vi "DataHandler Init.vi"(8 "error in (no error)":errorcluster, 11 "DataLogger in":refnum<class "DataLogger.lvclass">) -> (0 "error out":errorcluster, 3 "DataLogger out":refnum<class "DataLogger.lvclass">)   [LabVIEW 2020, in "Volatus.lvlib" / "DataLogger.lvclass"]
uses:
  DataLogger.lvclass
  C:/dev/lv20CE/relink/lv-volatus/Volatus/Task/Task.lvclass
  C:/Program Files (x86)/National Instruments/LabVIEW 2020/vi.lib/ActorFramework/Actor/Actor.lvclass
  LoggingIdentity/LoggingIdentity.lvclass
  C:/dev/lv20CE/relink/lv-volatus/Volatus/Identity/Identity.lvclass
  LoggingAPI/LoggingAPI.lvclass
  C:/dev/lv20CE/relink/lv-volatus/Volatus/API/API.lvclass
  Task/Task.lvclass/Task.ctl
  VolatusAPI/VolatusAPI.lvclass/VolatusAPI.ctl
  <vilib>/ActorFramework/Actor/Actor.lvclass/Actor.ctl
  <vilib>/ActorFramework/Message Enqueuer/Message Enqueuer.lvclass/Message Enqueuer.ctl
  DataLogger.lvclass/DataLogger.ctl
  <vilib>/ActorFramework/Message Enqueuer/Init from Existing Queue.vi
  Identity/Key.vi
  <vilib>/Utility/error.llb/Error Cluster From Error Code.vi
  API/API.lvclass
  <vilib>/ActorFramework/Message Enqueuer/Message Enqueuer.lvclass
  Identity/Identity.lvclass
  Task/Task.lvclass
  <vilib>/ActorFramework/Actor/Actor.lvclass
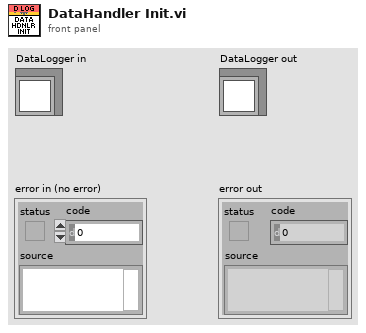
[diagram p1: front panel]
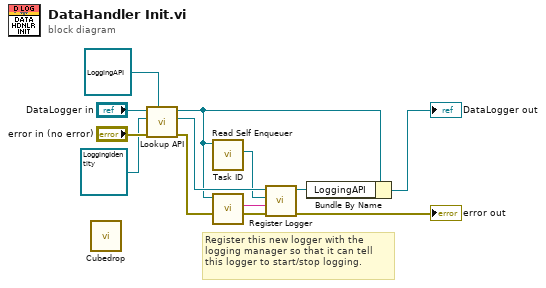
[diagram p0: block diagram]
diagram:
  # "Register this new logger with the logging manager so that it can tell this logger to start/stop logging."
  n1 = call "Cubedrop.vi"() -> ()  [unwired: 12 in]
  n2 = call "Lookup API.vi"("API Type"=refnum<class "LoggingAPI.lvclass"> refnum ("VolatusDataLogger:LoggingAPI.lvclass"), "error in (no error)"="error in (no error)", "Identity"=refnum<class "LoggingIdentity.lvclass"> refnum ("VolatusDataLogger:LoggingIdentity.lvclass"), "Task in"="DataLogger in") -> ("error out"=w5:errorcluster, "API"=w8:refnum<class "LoggingAPI.lvclass">, "Task out"=w2:refnum<class "DataLogger.lvclass">)  [unwired: 5 in]
  n3 = call <vilib>:"Read Self Enqueuer.vi"("Actor"=w2) -> ("Self Enqueuer"=w7:refnum<class "Message Enqueuer.lvclass">)  [unwired: 10 in]
  n4 = call-dynamic "Task ID.vi"("DataLogger in"=w2) -> ("Task ID"=w6:string)  [unwired: 8 in, 2 out]
  n5 = call "Register Logger.vi"("error in (no error)"=w5, "Task ID"=w6, "EnQr"=w7, "LoggingAPI in"=w8) -> ("error out"=→"error out":errorcluster, "LoggingAPI out"=w3:refnum<class "LoggingAPI.lvclass">)  [unwired: 6 in]
  n6 = Bundle By Name(cluster=w2, "LoggingAPI"=w3) -> (→"DataLogger out":refnum<class "DataLogger.lvclass">)
